vi "BasicReadoutV775.vi"() -> ()   [LabVIEW 2014]
uses:
  Program Files (x86)/CAEN/Comm/labview/CAENComm.lvlib
panel:
  in  "BLT?":bool
  out "Loop Counter":i32
  out "Event Counter":u32
  out "# Data":i32
  out "TDC Raw":u32[](array[numeric]) format="%.0b"
  out "QDC Raw":u32[](array[numeric]) format="%.0x"
  out "Results":T1(array[cluster]) {"GeoAddr" format="%.0x"}
  in  "stop":bool
  out "TDC Histogram":u16[](graph)
  out "error out":errorcluster
  in  "Channel for hist":u8=30
  out "Decode time":dbl
  in  "Low Range threshold":u16
  in  "VME Base Address":u32=4026597376 format="%.0x"
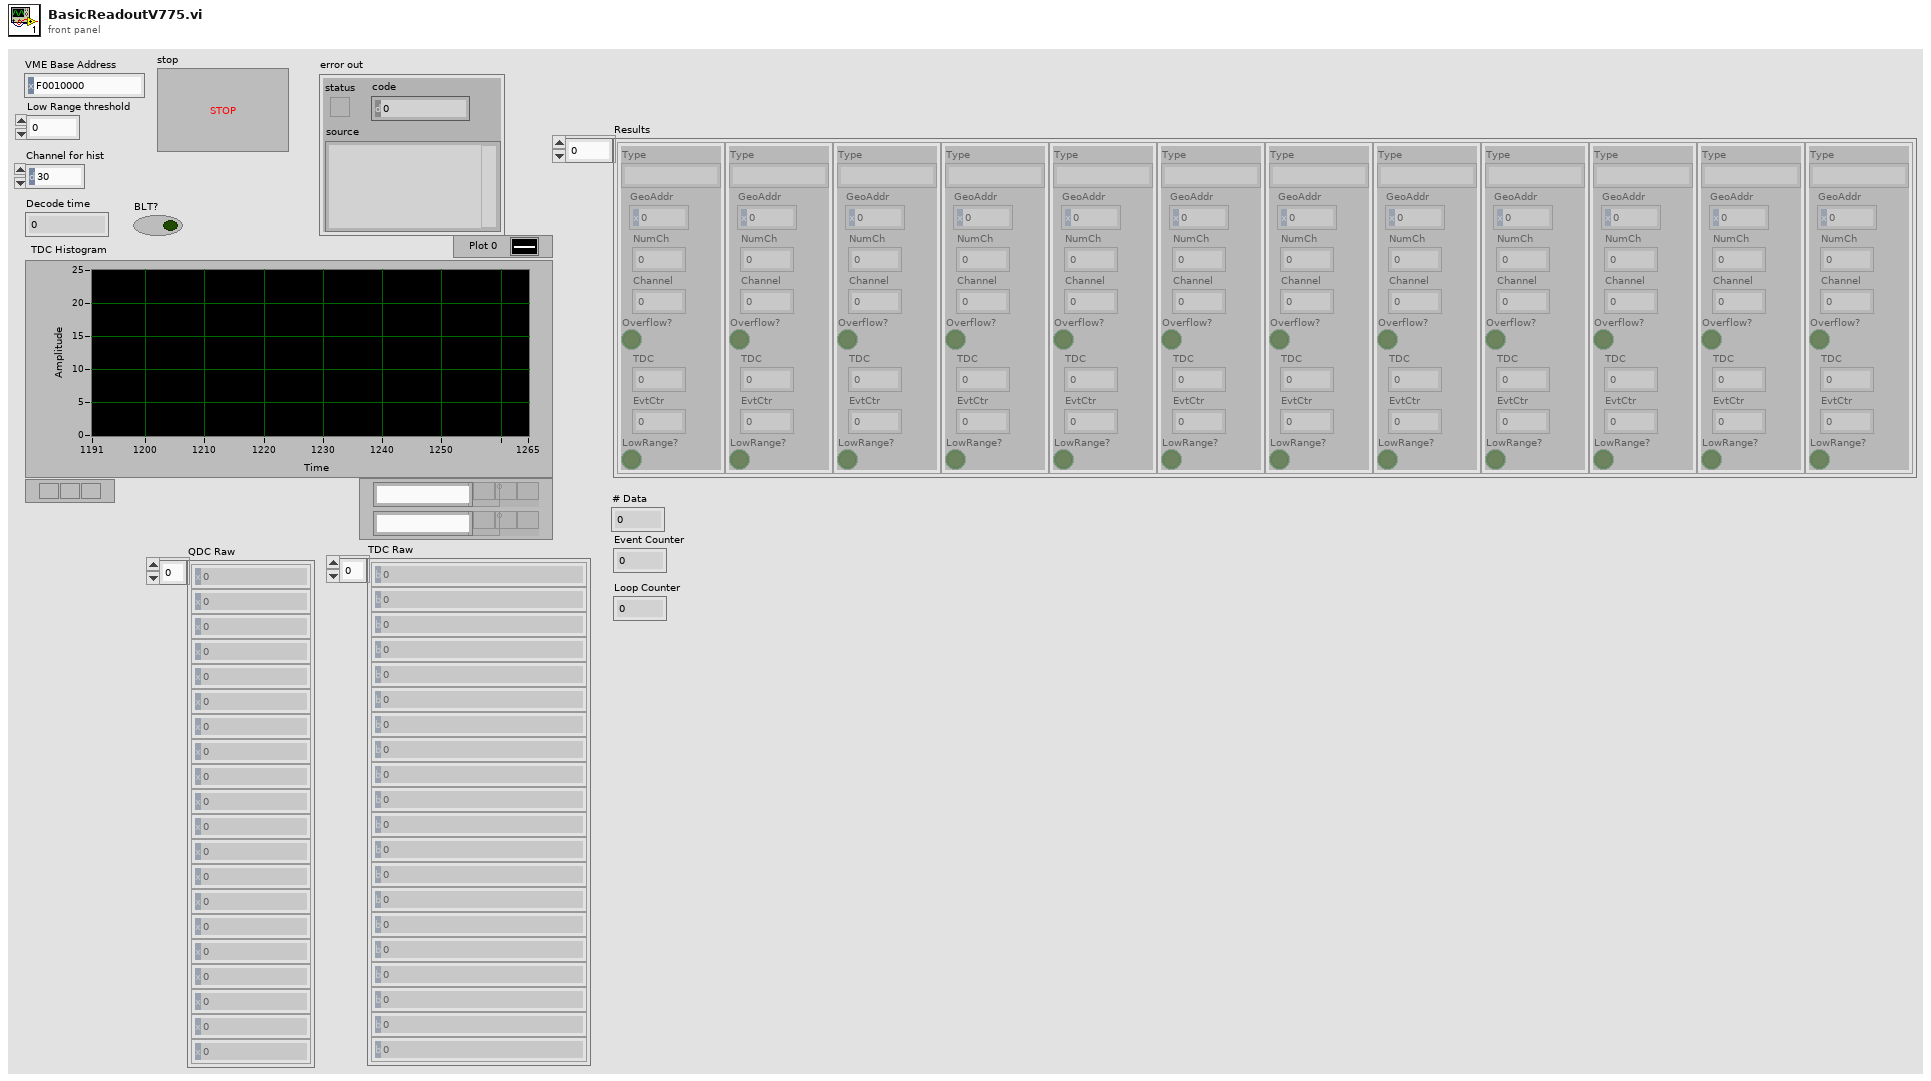
[diagram p1: front panel]
types:
  T1 = cluster{"Type":string, "GeoAddr":u8, "NumCh":u8, "Channel":u8, "Overflow?":bool, "TDC":u16, "EvtCtr":u32, "LowRange?":bool}[]
  T2 = cluster{"Type":string, "GeoAddr":u8, "NumCh":u8, "Channel":u8, "Overflow?":bool, "QDC":u16, "EvtCtr":u32, "Underflow?":bool}[]
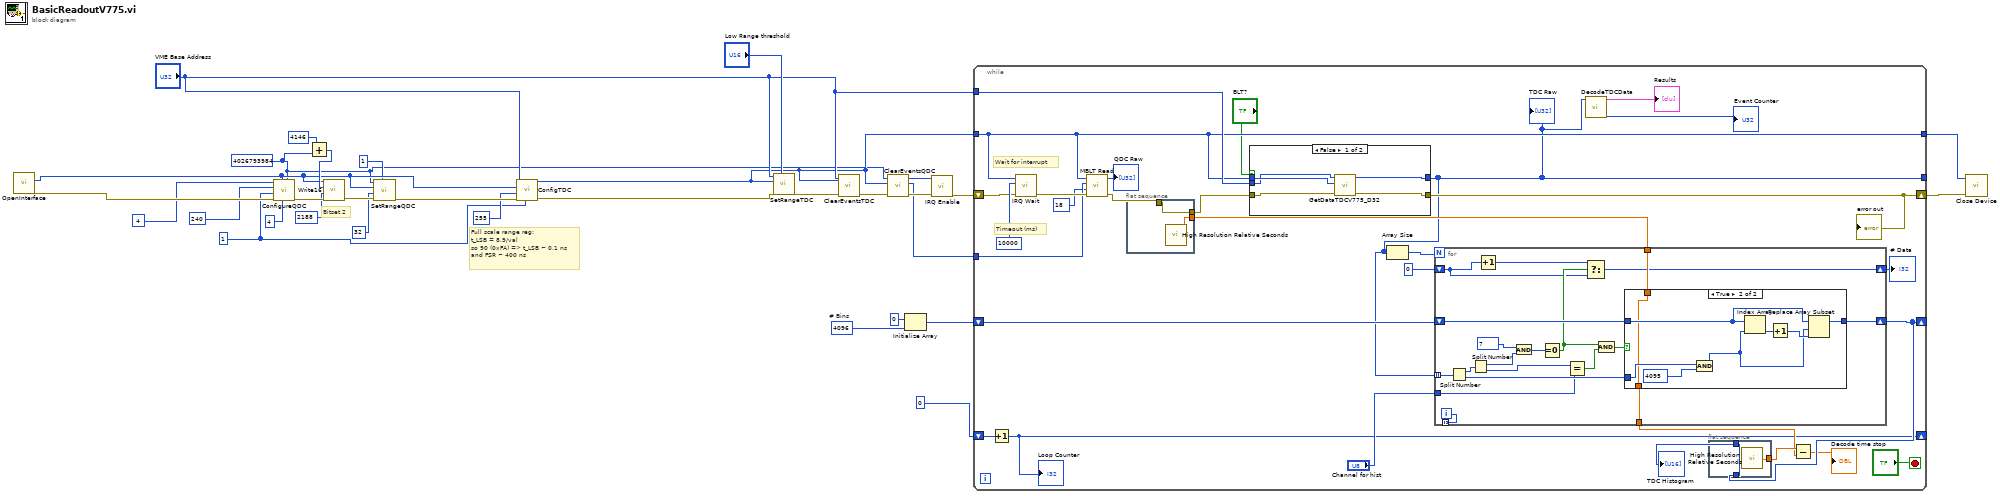
[diagram p0: block diagram]
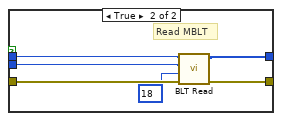
[diagram p2: hidden frame]
diagram:
  w2 = u16 1 ("# of events before transfer (max 32)")
  w4 = u32 4026793984 ("VME module Base Address")
  w27 = u16 4096  # # Bins
  # "Full scale range reg:\nt_LSB = 8.9/val\nso 90 (0xFA) => t_LSB ~ 0.1 ns\nand FSR ~ 400 ns"
  # "Bitset 2"
  n1 = call "OpenInterface.vi"() -> ("error out"=w22:errorcluster, "handle"=w12:i32)  [unwired: 9 in, 1 out]
  n2 = call "ConfigureQDC.vi"("VME module Base Address"=w4, "IRQ Lvl"=u16 4, "handle"=w12, "error in (no error)"=w22, "# of events before transfer (max 32)"=w2, "CBLT Addr"=u16 240, "Geo Addr"=u16 4) -> ("error out"=w18:errorcluster)  [unwired: 3 in, 1 out]
  n3 = Add(x=u32 4146, y=w4) -> (x+y=w16:u32)
  n4 = call "Write16.vi"("error in (no error)"=w18, "Data"=2188, "Address"=w16, "handle"=w12) -> ("error out"=w14:errorcluster)  [unwired: 7 in]
  n5 = call "SetRangeQDC.vi"("Low Range threshold"=u16 1, "error in (no error)"=w14, "High range threshold"=u16 32, "handle"=w12, "VME module Base Address"=w4) -> ("error out"=w13:errorcluster)  [unwired: 6 in]
  n6 = call "ConfigTDC.vi"("# Evts to Acquire"=w2, "error in (no error)"=w13, "FSR setting"=u16 255 ("Data"), "handle"=w12, "VME Base Address"="VME Base Address") -> ("error out"=w32:errorcluster, "handle out"=w7:i32)  [unwired: 5 in]
  n7 = call "SetRangeTDC.vi"("Low Range threshold"="Low Range threshold", "error in (no error)"=w32, "handle"=w7, "VME module Base Address"="VME Base Address") -> ("error out"=w30:errorcluster)  [unwired: 5 in, 2 out]
  n8 = call "ClearEventsTDC.vi"("error in (no error)"=w30, "handle"=w7, "VME module Base Address"="VME Base Address") -> ("error out"=w9:errorcluster)  [unwired: 6 in, 2 out]
  n9 = call "ClearEventsQDC.vi"("error in (no error)"=w9, "handle"=w7, "VME module Base Address"=w4) -> ("error out"=w8:errorcluster, "VME module Base Address out"=w5:u32, "handle out"=w6:i32)  [unwired: 6 in]
  n10 = Initialize Array(u16 0 ("element"), w27) -> (w29:u16[])
  n11 = call "IRQ Enable.vi"("error in (no error)"=w8, "handle"=w6) -> ("error out"=w26:errorcluster)  [unwired: 9 in]
  n12 = while {
    tunnel: "VME Base Address" -> [w36]
    tunnel: [w34] -> _
    shift-right: [w37] -> w24
    shift-left: w26 -> [w50]
    shift-right: [w57] -> _
    shift-left: w29 -> [w61]
    tunnel: w7 -> [w35]
    tunnel: [w35] -> w23
    tunnel: w5 -> [w48]
    shift-right: [w39] -> _
    shift-left: 0 -> [w40]
    stop <- "stop" stop-if-true
    # "Wait for interrupt"
    # "Timeout (ms)"
    n13 = Increment(x=w40) -> (x+1=w39:i32)
    "Loop Counter" <- w39
    n14 = call "IRQ Wait.vi"("error in (no error)"=w50, "Timeout"=u32 10000, "handle"=w35) -> ("error out"=w49:errorcluster)  [unwired: 8 in]
    n15 = call "MBLT Read.vi"("error in (no error)"=w49, "BltSize"=18, "Address"=w48, "handle"=w35) -> ("error out"=w46:errorcluster, "Buff"=→"QDC Raw":u32[])  [unwired: 5 in, 1 out]
    n16 = flat-sequence {
      tunnel: [w74] -> w38
      tunnel: w46 -> [w74]
      tunnel: [w73] -> w51
      frame #0 {
        n17 = call <vilib>:"High Resolution Relative Seconds.vi"() -> ("relative seconds"=w73:dbl)
      }
    }
    n18 = case shown="False" "BLT?" {
      tunnel: w38 -> [w64 w72]
      tunnel: [w66 w71] -> w37
      tunnel: w36 -> [w62 w69]
      tunnel: w35 -> [w63 w68]
      tunnel: [w65 w67] -> w34
      frame False {
        n19 = call "GetDataTDCV775_D32.vi"("error in (no error)"=w64, "handle in"=w63, "VME Base Address"=w62) -> ("error out"=w66:errorcluster, "Array"=w65:u32[])  [unwired: 6 in, 1 out]
      }
      frame True {
        # "Read MBLT"
        n20 = call "BLT Read.vi"("error in (no error)"=w72, "BltSize"=18, "Address"=w69, "handle"=w68) -> ("error out"=w71:errorcluster, "Buff"=w67:u32[])  [unwired: 5 in, 1 out]
      }
    }
    "error out" <- w37
    "TDC Raw" <- w34
    n21 = Array Size(array=w34) -> (size(s)=w52:i32)
    n22 = for {
      N: w52 -> [_]
      tunnel: w34 -> [w93] mode=indexing
      shift-right: [w84] -> w57
      shift-left: w61 -> [w85]
      tunnel: "Channel for hist" -> [w83]
      tunnel: w51 -> [w82]
      tunnel: [w81] -> w54
      shift-right: [w76] -> w42
      shift-left: 0 -> [w78]
      tunnel: [w75] -> _ mode=indexing
      i -> [w75]
      n23 = Split Number(x=w93) -> (hi(x)=w92:u16, lo(x)=w89:u16)
      n24 = Split Number(x=w92) -> (hi(x)=w88:u8, lo(x)=w80:u8)
      n25 = Increment(x=w78) -> (x+1=w77:i32)
      n26 = And(x=u8 7, y=w88) -> (x .and. y?=w90:u8)
      n27 = Equal To 0?(x=w90) -> (x = 0?=w79:bool)
      n28 = Equal?(x=w80, y=w83) -> (x = y?=w86:bool)
      n29 = Select(t=w77, s=w79, f=w78) -> (s? t:f=w76:i32)
      n30 = And(x=w79, y=w86) -> (x .and. y?=w87:bool)
      n31 = case shown="True" w87 {
        tunnel: w89 -> [_ w102]
        tunnel: w85 -> [w95 w100]
        tunnel: [w95 w98] -> w84
        tunnel: w82 -> [w94 w97]
        tunnel: [w94 w97] -> w81
        frame False {
        }
        frame True {
          n32 = And(x=w102, y=u16 4095) -> (x .and. y?=w96:u16)
          n33 = Index Array(array=w100, index=w96) -> (element=w101:u16)
          n34 = Increment(x=w101) -> (x+1=w99:u16)
          n35 = Replace Array Subset(array=w100, new element=w99, index=w96) -> (w98:u16[])
        }
      }
    }
    "# Data" <- w42
    n36 = call "DecodeTDCData.vi"("Buff"=w34) -> ("Event Counter"=→"Event Counter":u32, "Array"=→"Results":T2)  [unwired: 8 in, 1 out]
    n37 = flat-sequence {
      tunnel: w57 -> [w105]
      tunnel: [w105] -> w56
      tunnel: [w104] -> w55
      frame #0 {
        n38 = call <vilib>:"High Resolution Relative Seconds.vi"() -> ("relative seconds"=w104:dbl)
      }
    }
    n39 = Subtract(x=w55, y=w54) -> (x-y=→"Decode time":dbl)
    "TDC Histogram" <- w56
  }
  n40 = call "Close Device.vi"("error in (no error)"=w24, "handle"=w23) -> ()  [unwired: 9 in, 1 out]
